vi "readU16.vi"(8 "error in (no error)":errorcluster, 9 "Timeout":i32, 10 "NumberOfElements":u32, 11 "ModbusPort1ReadFIFO in":refnum<class "ModbusPort2ReadFIFO.lvclass">) -> (0 "error out":errorcluster, 1 "ElementsRemaining":u32, 2 "Data":u16[](array[numeric]), 3 "ModbusPort1ReadFIFO out":refnum<class "ModbusPort2ReadFIFO.lvclass">)   [LabVIEW 2015, in "ModbusPort2ReadFIFO.lvclass"]
uses:
  ModbusPort2ReadFIFO.lvclass
  ModbusPort2ReadFIFO.lvclass/ModbusPort2ReadFIFO.ctl
  <vilib>/Utility/error.llb/Error Cluster From Error Code.vi
  <vilib>/rvi/errors/niLvFpgaAdjustHostInterfaceError.vi
  <vilib>/rvi/interface/nirviMethod/nirviMethod.xnode
  <vilib>/FPGAPlugInAG/Dynamic/niLvFpga_ReadFifo_Dynamic.vi
  <vilib>/rvi/errors/niLvFpgaMergeErrorWithErrorCode.vi
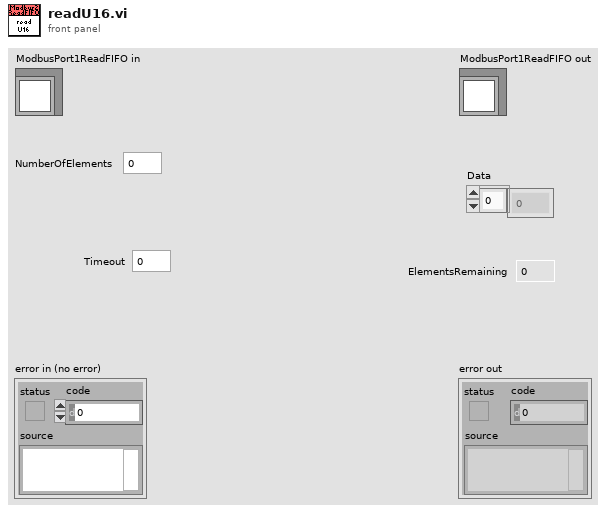
[diagram p1: front panel]
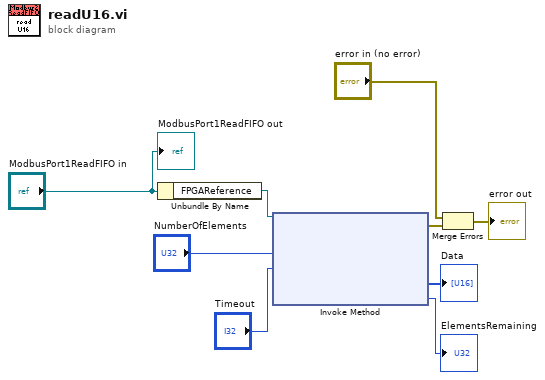
[diagram p0: block diagram]
diagram:
  n1 = Unbundle By Name("ModbusPort1ReadFIFO in") -> ("FPGAReference"=w1:refnum<k20>)
  n2 = xnode "Invoke Method"("FPGA VI Reference In"=w1, "Number of Elements"="NumberOfElements", "Timeout (ms)"="Timeout") -> ("error out"=w8:errorcluster, "Data"=→"Data":u16[], "Elements Remaining"=→"ElementsRemaining":u32)  [unwired: 1 in, 1 out]
  n3 = Merge Errors("error in (no error)", w8) -> (→"error out":errorcluster)
  "ModbusPort1ReadFIFO out" <- "ModbusPort1ReadFIFO in"
